vi "source_config.vi"(8 "error in (no error)":errorcluster, 11 "Input parameters":T1={"Measurement type"=enum."Debug", "Sensor type"=enum."HPK_8in_271ch", "Identifier"="test.txt", "Open after execution?"=FALSE, "Plot after execution?"=FALSE, "Display channel"=0, "Voltage Delay (s)"=0.5, "Switch Delay (s)"=0.01, "VISA resource name source"="", "VISA resource name DMM"="", "VISA resource name LCR"="", "Compliance  Level (A)"=10.0, "Voltage Limit (V)"=1000.0, "Data storage location"="", "Scan voltages"="", "Use source as DMM?"=FALSE, "LCR signal frequenzy (Hz)"=10.0, "DMM device"=enum."Keithley2001", "Sampling number"=1, "Use env. sensors on"=enum."Sensirion sht1x/7x", "Switchboard Handle"=0, "Use Switchboard"=FALSE, "LCR signal voltage (V)"=10000.0, "Repeat"=1, "Scan voltages IV"="", "Scan voltages CV"="", "Hex pad numbers?"=FALSE, "Set measurement type"=enum."Debug", "Custom pad scan"="", "IV voltage Delay (s)"=0.5, "CV voltage Delay (s)"=0.5, "Needle measurement?"=FALSE, "Comments"="test.txt", "LCR signal frequenzy (kHz)"=10.0, "Compliance  Level (uA)"=10.0, "Open Correction Array"=array2304x3[6912 elements], "Current set voltage"=0.0, "Last set voltage"=0.0, "Current channel"=0, "Last OpenCorrection index"=-1, "Total curr/vltg every x steps"=10, "Current channel iteration"=0, "No CV corrections"=FALSE, "Mapfile"="", "Corrfile"="", "IV voltage file"=path "", "CV voltage file"=path "", "IV Switch Delay (s)"=0.01, "CV Switch Delay (s)"=0.01, "Invert polarity"=FALSE, "Set debug dirs"=FALSE, "Is n on p"=FALSE, "Source interlock?"=TRUE, "Voltage file used?"=FALSE, "Pad mask"="", "Mask pad above (uA)"=1.0, "LCR device"=enum."LCR_E4980", "Source device"=enum."Source_2410"} {"CV Switch Delay (s)" format="%#_13g"; "IV Switch Delay (s)" format="%#_13g"; "Last set voltage" format="%#_13g"; "Current set voltage" format="%#_13g"; "CV voltage Delay (s)" format="%#_13g"; "IV voltage Delay (s)" format="%#_13g"; "Voltage Limit (V)" format="%#_13g"; "Voltage Delay (s)" format="%#_13g"; "Switch Delay (s)" format="%#_13g"}) -> (0 "error out":errorcluster, 2 "Output Level (0)":dbl, 3 "VISA resource name out":refnum<visa-resource-name>)   [LabVIEW 2016]
doc: "Sets configuration for source meter."
uses:
  input_params.ctl
  <instrlib>/Keithley 24XX/Keithley 24XX.lvlib
  <instrlib>/Keithley 648X Series/Keithley 648X Series.lvlib
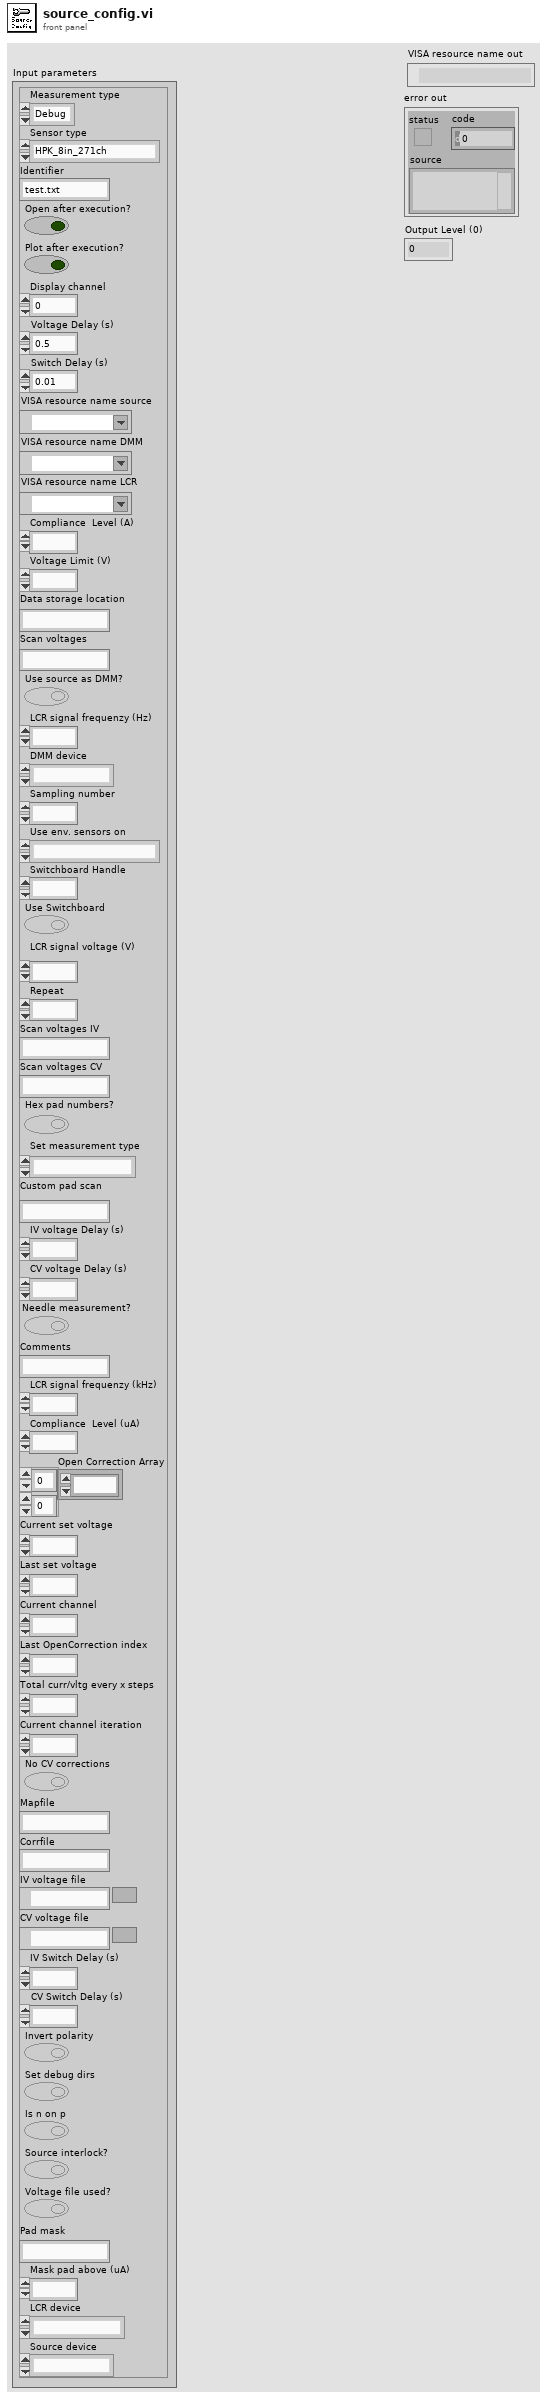
[diagram p1: front panel]
types:
  T1 = typedef "input_params.ctl" = cluster{"Measurement type":enum16{"IV", "CV", "Debug", "Test_contact"}, "Sensor type":enum16{"HPK_6in_135ch", "HPK_8in_271ch", "IFX_8in_256ch", "Diode", "HPK_6in_239ch", "Full_Matrix", "HPK_8in_271ch_full", "HPK_8in_198ch", "LumiCal"}, "Identifier":string, "Open after execution?":bool, "Plot after execution?":bool, "Display channel":i32, "Voltage Delay (s)":dbl, "Switch Delay (s)":dbl, "VISA resource name source":refnum<visa-resource-name>, "VISA resource name DMM":refnum<visa-resource-name>, "VISA resource name LCR":refnum<visa-resource-name>, "Compliance  Level (A)":dbl, "Voltage Limit (V)":dbl, "Data storage location":string, "Scan voltages":string, "Use source as DMM?":bool, "LCR signal frequenzy (Hz)":dbl, "DMM device":enum16{"Keithley2001", "Keithley2450", "Keithley2410", "Keithley6485", "Keithley6487", "Keithley6517"}, "Sampling number":i32, "Use env. sensors on":enum16{"Sensirion sht1x/7x", "Switch Matrix", "Probecard"}, "Switchboard Handle":u32, "Use Switchboard":bool, "LCR signal voltage (V)":dbl, "Repeat":i32, "Scan voltages IV":string, "Scan voltages CV":string, "Hex pad numbers?":bool, "Set measurement type":enum16{"IV", "CV", "Debug", "Test_contact", "IV+CV"}, "Custom pad scan":string, "IV voltage Delay (s)":dbl, "CV voltage Delay (s)":dbl, "Needle measurement?":bool, "Comments":string, "LCR signal frequenzy (kHz)":dbl, "Compliance  Level (uA)":dbl, "Open Correction Array":dbl[][], "Current set voltage":dbl, "Last set voltage":dbl, "Current channel":i32, "Last OpenCorrection index":i32, "Total curr/vltg every x steps":i32, "Current channel iteration":i32, "No CV corrections":bool, "Mapfile":string, "Corrfile":string, "IV voltage file":path, "CV voltage file":path, "IV Switch Delay (s)":dbl, "CV Switch Delay (s)":dbl, "Invert polarity":bool, "Set debug dirs":bool, "Is n on p":bool, "Source interlock?":bool, "Voltage file used?":bool, "Pad mask":string, "Mask pad above (uA)":dbl, "LCR device":enum16{"LCR_E4980", "AGILENT_4263X"}, "Source device":enum16{"Source_2410", "Source_6487"}}
  T2 = cluster{"Baud Rate":u32, "Parity":u16, "Data Bits":u16, "Stop Bits":u16, "Flow Control":u16}
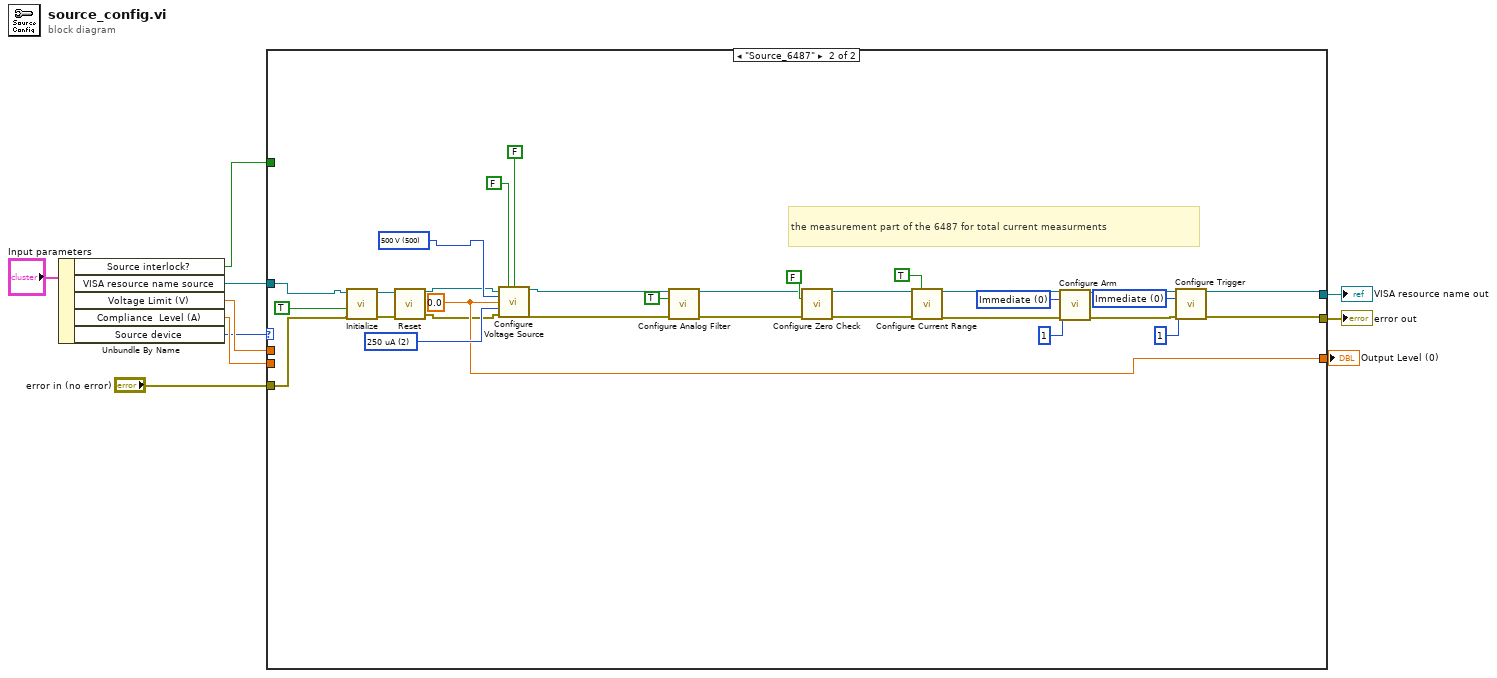
[diagram p0: block diagram]
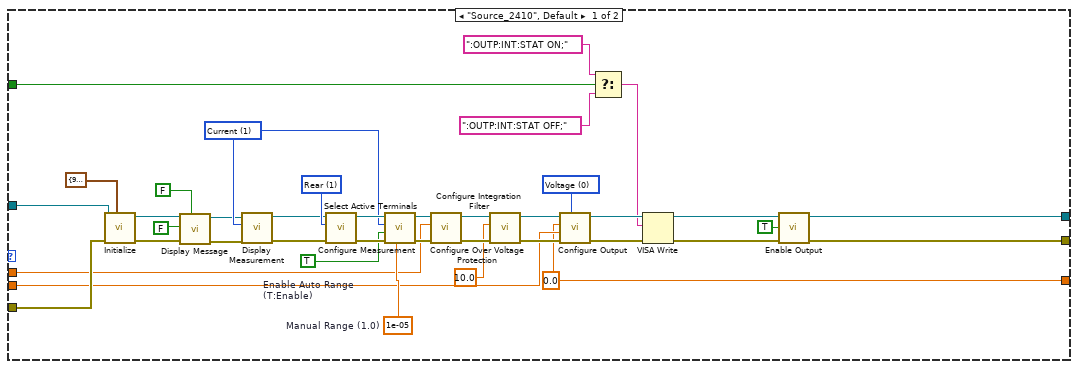
[diagram p2: hidden frame]
diagram:
  n1 = Unbundle By Name("Input parameters") -> ("Source interlock?"=w8:bool, "VISA resource name source"=w7:refnum<visa-resource-name>, "Voltage Limit (V)"=w6:dbl, "Compliance  Level (A)"=w5:dbl, "Source device"=w2:enum16{"Source_2410", "Source_6487"})
  n2 = case shown="\"Source_6487\"" w2 {
    tunnel: "error in (no error)" -> [w45 w79]
    tunnel: w8 -> [w23 _]
    tunnel: w7 -> [w19 w80]
    tunnel: w6 -> [w18 _]
    tunnel: w5 -> [w17 _]
    tunnel: [w13 w50] -> w4
    tunnel: [w14 w51] -> w3
    tunnel: [w15 w73] -> w1
    frame "Source_2410", Default {
      w33 = 1e-05  # Manual Range (1.0)
      w34 = TRUE  # Enable Auto Range (T:Enable)
      w32 = u16 1 items=["Voltage", "Current", "Resistance"] ("Displayed Measurement (0: Voltage)")
      w42 = u16 1 items=["Front", "Rear"] ("Active Terminals (0: Front)")
      w15 = 0.0 ("Output Level (0)")
      w48 = u16 0 items=["Voltage", "Current"] ("Source Mode  (0: Voltage)")
      n3 = call <instrlib>:"Initialize.vi"("Serial Configuration"=T2 {"Baud Rate"=9600, "Parity"=0, "Data Bits"=8, "Stop Bits"=10, "Flow Control"=0}, "error in (no error)"=w45, "VISA resource name"=w19) -> ("error out"=w30:errorcluster, "VISA resource name out"=w31:refnum<visa-resource-name>)  [unwired: 7 in]
      n4 = call <instrlib>:"Display Message.vi"("Enable Lower Message (T: Enable)"=FALSE, "Enable Upper Message (T: Enable)"=FALSE, "error in (no error)"=w30, "VISA resource name"=w31) -> ("error out"=w29:errorcluster, "VISA resource name out"=w28:refnum<visa-resource-name>)  [unwired: 6 in]
      n5 = call <instrlib>:"Display Measurement.vi"("error in (no error)"=w29, "Displayed Measurement (0: Voltage)"=w32, "VISA resource name"=w28) -> ("error out"=w41:errorcluster, "VISA resource name out"=w40:refnum<visa-resource-name>)  [unwired: 7 in]
      n6 = call <instrlib>:"Select Active Terminals.vi"("error in (no error)"=w41, "Active Terminals (0: Front)"=w42, "VISA resource name"=w40) -> ("error out"=w43:errorcluster, "VISA resource name out"=w44:refnum<visa-resource-name>)  [unwired: 7 in]
      n7 = call <instrlib>:"Configure Measurement.vi"("Manual Range (1.0)"=w33, "error in (no error)"=w43, "Enable Auto Range (T:Enable)"=w34, "Function (0: Volts)"=w32, "VISA resource name"=w44) -> ("error out"=w46:errorcluster, "VISA resource name out"=w47:refnum<visa-resource-name>)  [unwired: 5 in]
      n8 = call <instrlib>:"Configure Over Voltage Protection.vi"("error in (no error)"=w46, "Voltage Limit (0.0 V)"=w18, "VISA resource name"=w47) -> ("error out"=w38:errorcluster, "VISA resource name out"=w39:refnum<visa-resource-name>)  [unwired: 7 in]
      n9 = call <instrlib>:"Configure Integration Filter.vi"("error in (no error)"=w38, "Measurement Speed (1 PLC)"=10.0, "VISA resource name"=w39) -> ("error out"=w37:errorcluster, "VISA resource name out"=w36:refnum<visa-resource-name>)  [unwired: 7 in]
      n10 = call <instrlib>:"Configure Output.vi"("Source Mode  (0: Voltage)"=w48, "error in (no error)"=w37, "Compliance  Level (0.1)"=w17, "Output Level (0)"=w15, "VISA resource name"=w36) -> ("error out"=w25:errorcluster, "VISA resource name out"=w24:refnum<visa-resource-name>)  [unwired: 5 in]
      n11 = Select(t=":OUTP:INT:STAT ON;" ("write buffer"), s=w23, f=":OUTP:INT:STAT OFF;" ("write buffer")) -> (s? t:f=w20:string)
      n12 = VISA Write(VISA resource name=w24, write buffer=w20, error in (no error)=w25) -> (VISA resource name out=w12:refnum<visa-resource-name>, error out=w11:errorcluster)  [unwired: 1 out]
      n13 = call <instrlib>:"Enable Output.vi"("error in (no error)"=w11, "Enable Output (T: Enable)"=TRUE ("Enable Output"), "VISA resource name"=w12) -> ("error out"=w13:errorcluster, "VISA resource name out"=w14:refnum<visa-resource-name>)  [unwired: 7 in]
    }
    frame "Source_6487" {
      w59 = u16 0 items=["Immediate", "Tlink"] ("Trigger Source (0: Immediate)")
      w61 = u16 0 items=["Immediate", "Timer", "Bus", "Tlink", "Manual", "Negative SOT", "Positive SOT", "Bidirectional SOT"] ("Arm Source (0: Immediate)")
      w73 = 0.0 ("Voltage Level (0 V)")
      w76 = u16 2 items=["25 mA", "2.5 mA", "250 uA", "25 uA"] ("Current Limit (25 mA)")
      w77 = u16 500 items=["10 V"=10, "50 V"=50, "500 V"=500] ("Voltage Source Range (10 V)")
      # "the measurement part of the 6487 for total current measurments"
      n14 = call <instrlib>:"Initialize.vi"("error in (no error)"=w79, "Reset (True)"=TRUE, "VISA resource name"=w80) -> ("error out"=w56:errorcluster, "VISA resource name out"=w57:refnum<visa-resource-name>)  [unwired: 7 in]
      n15 = call <instrlib>:"Reset.vi"("VISA resource name"=w57, "error in (no error)"=w56) -> ("VISA resource name out"=w55:refnum<visa-resource-name>, "error out"=w54:errorcluster)  [unwired: 12 in]
      n16 = call <instrlib>:"Configure Voltage Source.vi"("VISA resource name"=w55, "Enable Voltage Source (F: Disable)"=FALSE, "Enable Interlock (F: Disable)"=FALSE, "Voltage Source Range (10 V)"=w77, "Voltage Level (0 V)"=w73, "Current Limit (25 mA)"=w76, "error in (no error)"=w54) -> ("VISA resource name out"=w72:refnum<visa-resource-name>, "error out"=w71:errorcluster)  [unwired: 7 in]
      n17 = call <instrlib>:"Configure Analog Filter.vi"("VISA resource name"=w72, "Enable Damping Filter (T: Enable)"=TRUE, "error in (no error)"=w71) -> ("VISA resource name out"=w53:refnum<visa-resource-name>, "error out"=w52:errorcluster)  [unwired: 11 in]
      n18 = call <instrlib>:"Configure Zero Check.vi"("VISA resource name"=w53, "Enable Zero Check (T: Enable)"=FALSE ("Autozero"), "error in (no error)"=w52) -> ("VISA resource name out"=w67:refnum<visa-resource-name>, "error out"=w66:errorcluster)  [unwired: 11 in]
      n19 = call <instrlib>:"Configure Current Range.vi"("VISA resource name"=w67, "Autorange (T: Enable)"=TRUE, "error in (no error)"=w66) -> ("VISA resource name out"=w65:refnum<visa-resource-name>, "error out"=w62:errorcluster)  [unwired: 11 in]
      n20 = call <instrlib>:"Configure Arm.vi"("VISA resource name"=w65, "Arm Source (0: Immediate)"=w61, "Arm Loop Count (1)"=1, "error in (no error)"=w62) -> ("VISA resource name out"=w64:refnum<visa-resource-name>, "error out"=w63:errorcluster)  [unwired: 10 in]
      n21 = call <instrlib>:"Configure Trigger.vi"("VISA resource name"=w64, "Trigger Source (0: Immediate)"=w59, "Trigger Loop Count (1)"=1, "error in (no error)"=w63) -> ("VISA resource name out"=w51:refnum<visa-resource-name>, "error out"=w50:errorcluster)  [unwired: 10 in]
    }
  }
  "VISA resource name out" <- w3
  "error out" <- w4
  "Output Level (0)" <- w1
